vi "interpoldation.vi"() -> ()   [LabVIEW 2020]
uses:
  common/record_file_handler/VFH-file_cluster-r140_water.ctl
  common/record_file_handler/VFH-file_cluster-NanoVNA.ctl
  common/record_file_handler/VFH-VNA_File_Handler.lvlib
  <vilib>/gmath/NI_Gmath.lvlib
panel:
  out "X":dbl[](array[numeric]) format="%_6g"
  out "xi used":dbl[](array[numeric]) format="%_6g"
  out "XY Graph 3":cluster{"xi used":dbl[], "yi":dbl[]}[](graph)
  out "XY Graph 2":cluster{"Frequency":dbl[], "Permativity'":dbl[]}(graph)
  out "Waveform Graph 5":dbl[](graph)
  out "Waveform Graph 4":dbl[](graph)
  out "Waveform Graph 3":dbl[](graph)
  out "Waveform Graph 2":dbl[](graph)
  out "XY Graph":cluster{"Frequency":dbl[], "Permativity'":dbl[]}(graph)
  out "Waveform Graph":dbl[](graph)
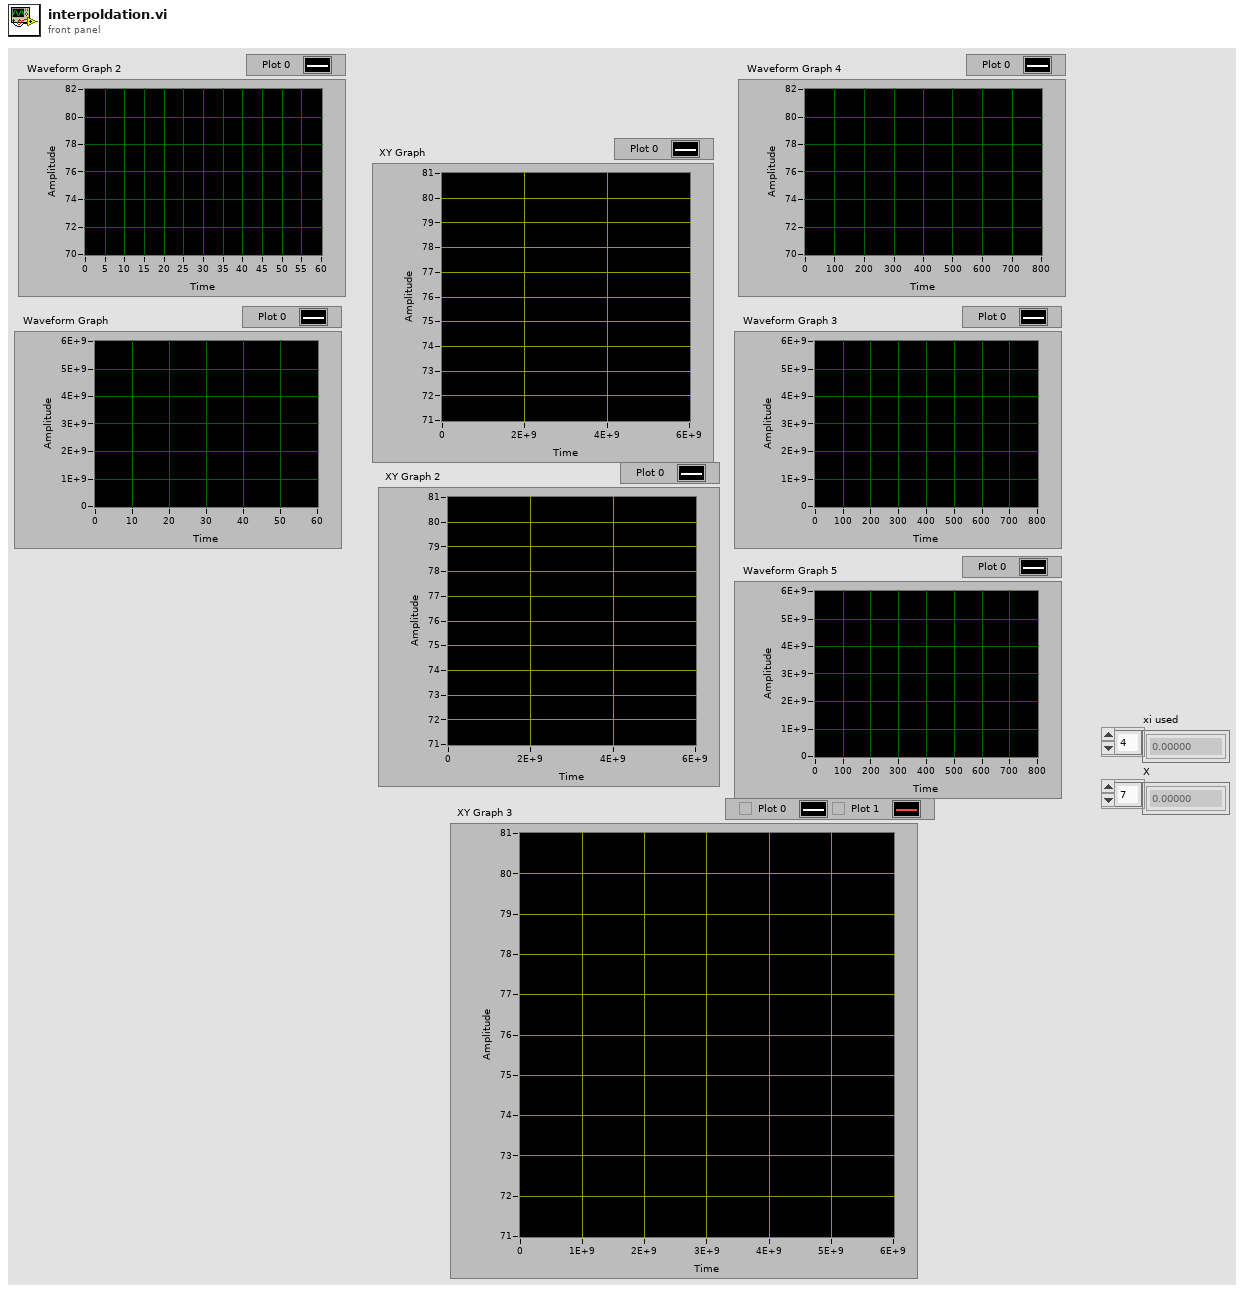
[diagram p1: front panel]
types:
  T1 = typedef "VFH-VNA_File_Handler.lvlib/VFH-file_cluster-NanoVNA.ctl" = cluster{"Frequency":dbl[], "S11_Real":dbl[], "S11_Imag":dbl[], "S21_Real":dbl[], "S21_Imag":dbl[], "S12_Real":dbl[], "S12_Imag":dbl[], "S22_Real":dbl[], "S22_Imag":dbl[]}
  T2 = typedef "VFH-VNA_File_Handler.lvlib/VFH-file_cluster-r140_water.ctl" = cluster{"Frequency":dbl[], "Permativity'":dbl[], "Q [S/m]":dbl[]}
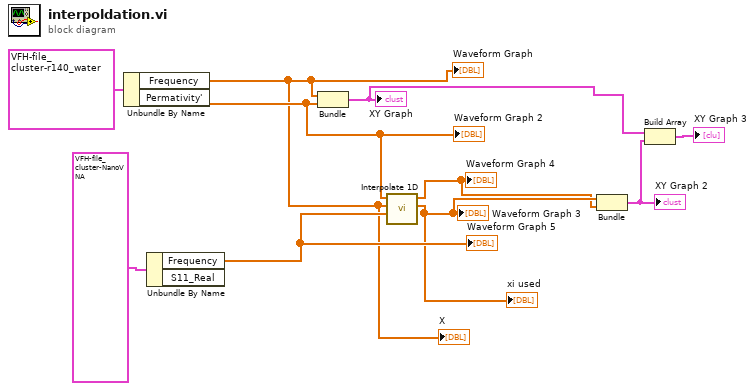
[diagram p0: block diagram]
diagram:
  n1 = Unbundle By Name(T2 {"Frequency"=[0.0, 100000000.0, 200000000.0, 300000000.0, 400000000.0, 500000000.0, 600000000.0, 700000000.0, 800000000.0, 900000000.0, 1000000000.0, 1100000000.0, 1200000000.0, 1300000000.0, 1400000000.0, 1500000000.0, 1600000000.0, 1700000000.0, 1800000000.0, 1900000000.0, 2000000000.0, 2100000000.0, 2200000000.0, 2300000000.0, 2400000000.0, 2500000000.0, 2600000000.0, 2700000000.0, 2800000000.0, 2900000000.0, 3000000000.0, 3100000000.0, 3200000000.0, 3300000000.0, 3400000000.0, 3500000000.0, 3600000000.0, 3700000000.0, 3800000000.0, 3900000000.0, 4000000000.0, 4100000000.0, 4200000000.0, 4300000000.0, 4400000000.0, 4500000000.0, 4600000000.0, 4700000000.0, 4800000000.0, 4900000000.0, 5000000000.0, 5100000000.0, 5200000000.0, 5300000000.0, 5400000000.0, 5500000000.0, 5600000000.0, 5700000000.0, 5800000000.0, 5900000000.0], "Permativity'"=[80.946, 80.94304, 80.93418, 80.9194, 80.89869999999999, 80.87214, 80.83967999999999, 80.8014, 80.75724, 80.70721999999999, 80.65147999999999, 80.58992, 80.52264, 80.44964, 80.37096, 80.28664, 80.19669999999999, 80.10122000000001, 80.00026, 79.89376, 79.78192, 79.66468, 79.54214, 79.4143, 79.28126, 79.14316000000001, 78.99994000000001, 78.85166, 78.69846, 78.54038, 78.37748, 78.2099, 78.03757999999999, 77.86072, 77.67931999999999, 77.49346, 77.30326, 77.1087, 76.90998, 76.70714, 76.50018, 76.28934000000001, 76.07464, 75.85604, 75.63382, 75.40794, 75.17848000000001, 74.9456, 74.70927999999999, 74.46979999999999, 74.227, 73.98114000000001, 73.73226, 73.48046, 73.22576, 72.96834000000001, 72.70824, 72.44554000000001, 72.1803, 71.91266], "Q [S/m]"=[0.0, 0.0026161179999999997, 0.010463222000000001, 0.023537540000000003, 0.0418329, 0.06534054, 0.09404924, 0.1279454, 0.167013, 0.2112338, 0.2605864, 0.3150476, 0.37459159999999997, 0.4391914, 0.5088154, 0.583433, 0.6630076, 0.7475032, 0.8368807999999999, 0.9310994000000001, 1.0301156, 1.1338840000000001, 1.2423579999999999, 1.35549, 1.473228, 1.5955240000000002, 1.7223160000000002, 1.8535499999999998, 1.989176, 2.129124, 2.273342, 2.4217579999999996, 2.574326, 2.730966, 2.8916180000000002, 3.056212, 3.224694, 3.396974, 3.572996, 3.752688, 3.9359719999999996, 4.122786, 4.313048, 4.50668, 4.703626, 4.903792, 5.107122, 5.313518, 5.522921999999999, 5.735254, 5.950438, 6.1683900000000005, 6.389044, 6.612316, 6.83813, 7.066416, 7.2971, 7.5300899999999995, 7.765326, 8.002728000000001]} ("Water Cluster")) -> ("Frequency"=w1:dbl[], "Permativity'"=w10:dbl[])
  "Waveform Graph" <- w1
  "Waveform Graph 2" <- w10
  "X" <- w1
  n2 = Unbundle By Name(T1 {"Frequency"=array[801 elements], "S11_Real"=array[801 elements], "S11_Imag"=array[801 elements], "S21_Real"=array[801 elements], "S21_Imag"=array[801 elements], "S12_Real"=array[801 elements], "S12_Imag"=array[801 elements], "S22_Real"=array[801 elements], "S22_Imag"=array[801 elements]} ("avg output")) -> ("Frequency"=w7:dbl[])  [unwired: 1 out]
  "Waveform Graph 5" <- w7
  n3 = Bundle("Frequency"=w1, "Permativity'"=w10) -> (w3:cluster{"Frequency":dbl[], "Permativity'":dbl[]})  [unwired: 1 in]
  "XY Graph" <- w3
  n4 = call <vilib>:"Interpolate 1D.vi"("xi"=w7, "X"=w1, "Y"=w10) -> ("xi used"=w6:dbl[], "yi"=w5:dbl[])  [unwired: 6 in, 1 out]
  "Waveform Graph 3" <- w6
  "Waveform Graph 4" <- w5
  "xi used" <- w6
  n5 = Bundle("xi used"=w6, "yi"=w5) -> (w4:cluster{"xi used":dbl[], "yi":dbl[]})  [unwired: 1 in]
  "XY Graph 2" <- w4
  n6 = Build Array(w3, w4) -> (→"XY Graph 3":cluster{"xi used":dbl[], "yi":dbl[]}[])
